vi "Decode Multiple.vi"   [LabVIEW 2020, in "feature_detection.lvlib" / "QR Code Detector.lvclass"]
doc: "Decode Multiple QR Codes in an image at the locations specified."
uses:
  QR Code Detector.lvclass
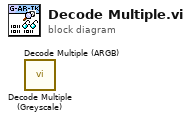
[diagram p0: block diagram]
diagram:
  n1 = call "Decode Multiple (Greyscale).vi"() -> ()  [unwired: 9 in, 3 out]
  n2 = call "Decode Multiple (ARGB).vi"() -> ()  [unwired: 9 in, 3 out]
